vi "4 channel - main interface.vi"() -> ()   [LabVIEW 2023]
uses:
  <vilib>/DAQmx/read.llb/DAQmx Read (Digital 1D Bool 1Chan 1Samp).vi
  <vilib>/DAQmx/create/channels.llb/DAQmx Create Channel (DI-Digital Input).vi
  Shared variables/exp.list.vi
  Shared variables/log.list.vi
  <vilib>/DAQmx/miscellaneous.llb/DAQmx Fill In Error Info.vi
  Shared variables/log.lvlib
panel:
  in  "main interface":T1(tab)
  in  "stop":bool
  in  "Manual control":bool
  in  "Channel":i8=1
  in  "Status":T2(ring)
  out "Current index":i8
  in  "add":bool
  in  "add to exp.list":dbl[](array[numeric])
  in  "Initial index":i8
  out "worker4 times":i8
  out "worker4 entry":i32
  out "worker4 status":dbl(slide) scale=0.0..100.0
  out "worker3 times":i8
  out "worker3 entry":i32
  out "worker3 status":dbl(slide) scale=0.0..100.0
  in  "worker2 on/off":bool
  out "Done":bool
  out "worker2 entry":i32
  out "worker1 entry":i32
  out "worker2 times":i8
  out "worker1 times":i8
  out "worker2 status":dbl(slide) scale=0.0..100.0
  out "worker1 status":dbl(slide) scale=0.0..100.0
  out "wash needle":bool
  out "sensor":bool[](array[boolean])
  in  "worker1 on/off":bool
  in  "worker3 on/off":bool
  in  "worker4 on/off":bool
  out "exp.list":string[][](array[string])
  out "log.list":string[][](array[string])
  # "Designed by @Xian Zheng"
  # "Designed by @Xian Zheng"
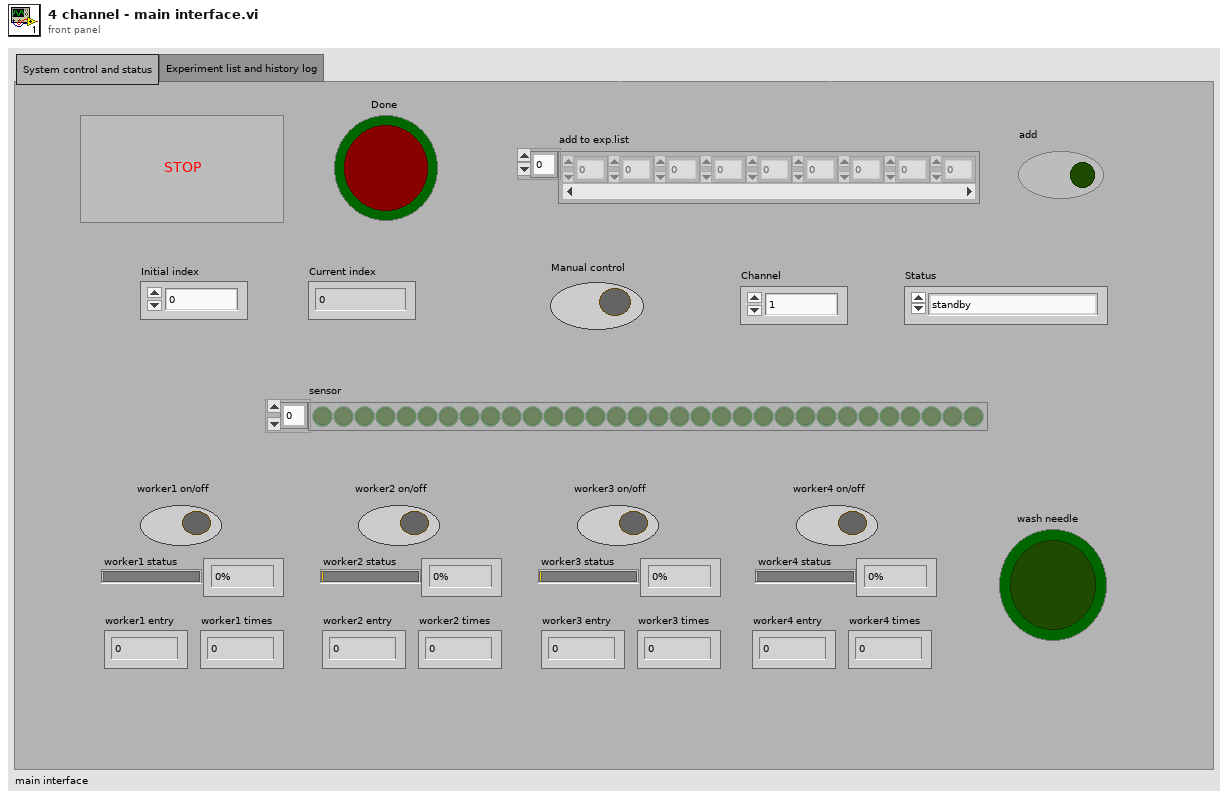
[diagram p1: front panel]
types:
  T1 = enum32{"System control and status", "Experiment list and history log"}
  T2 = enum16{"standby", "prepare droplet", "wash needle", "wash reactor", "wash sample loop", "deliver droplet", "offload product", "oscillate", "transfer product"}
  T3 = enum16{"check", "scan", "index", "read", "add", "write"}
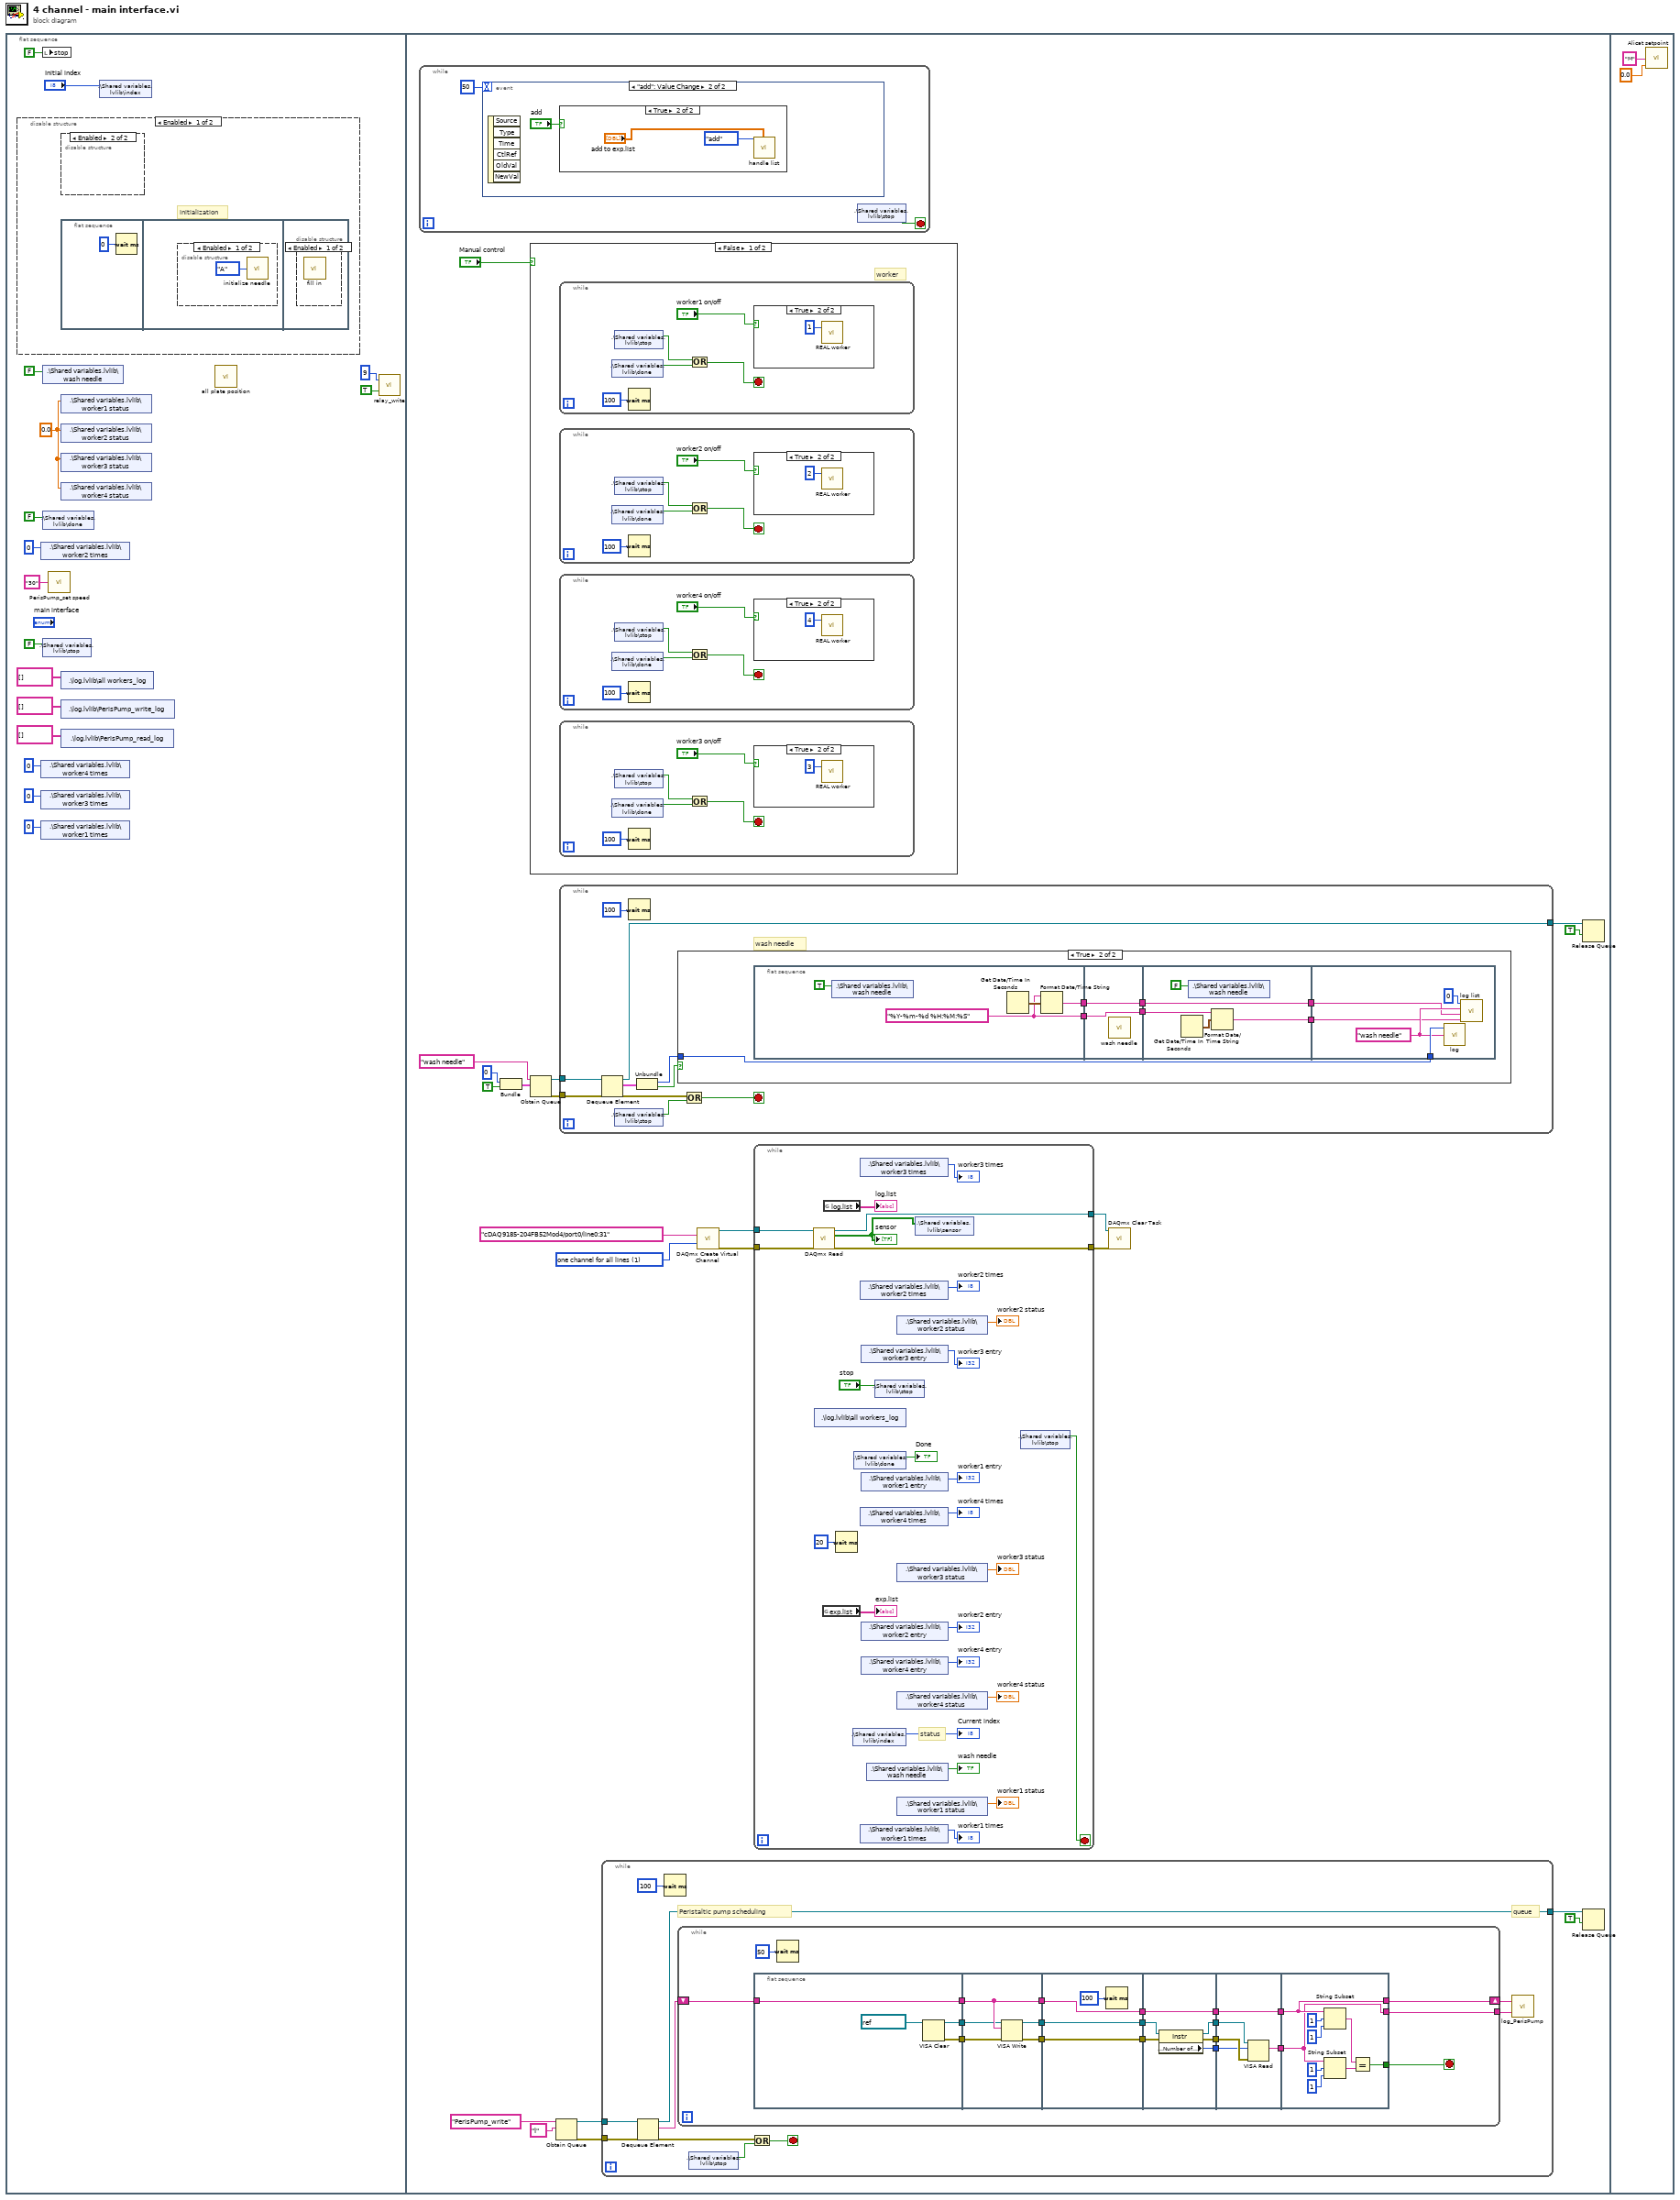
[diagram p0: block diagram]
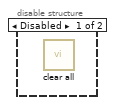
[diagram p2: hidden frame]
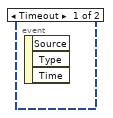
[diagram p6: hidden frame]
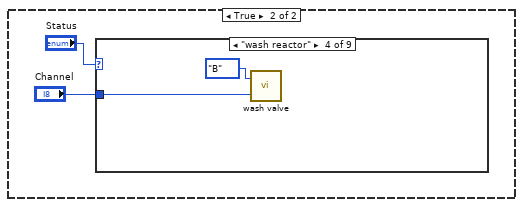
[diagram p13: hidden frame]
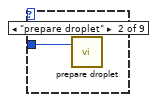
[diagram p15: hidden frame]
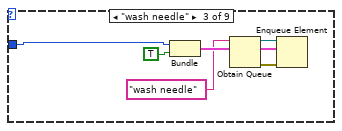
[diagram p16: hidden frame]
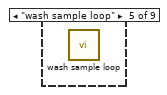
[diagram p17: hidden frame]
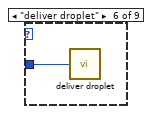
[diagram p18: hidden frame]
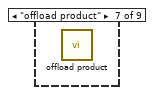
[diagram p19: hidden frame]
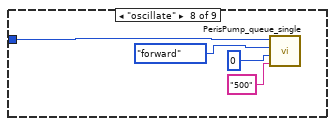
[diagram p20: hidden frame]
diagram:
  n1 = flat-sequence {
    frame #0 {
      w3 = 0.0 ("worker1 status")
      n2 = disable-structure shown="Enabled" {
        frame Enabled {
          # "initialization"
          n3 = disable-structure shown="Enabled" {
            frame Disabled {
              n4 = call "clear all.vi"() -> ()  [unwired: 12 in]
            }
            frame Enabled {
            }
          }
          n5 = flat-sequence {
            frame #0 {
              n6 = Wait (ms)(milliseconds to wait=u32 0) -> ()  [unwired: 1 out]
            }
            frame #1 {
              n7 = disable-structure shown="Enabled" {
                frame Enabled {
                  n8 = call "initialize needle.vi"("Switch to (A/B)"=enum16{"A", "B"}."A") -> ()  [unwired: 1 in]
                }
                frame Disabled {
                }
              }
            }
            frame #2 {
              n9 = disable-structure shown="Enabled" {
                frame Enabled {
                  n10 = call "fill in.vi"() -> ()  [unwired: 12 in]
                }
                frame Disabled {
                }
              }
            }
          }
        }
        frame Disabled {
        }
      }
      n11 = shared-variable ".\\Shared variables.lvlib\\worker2 times"(i8 0 ("worker1 times")) -> ()  [unwired: 1 in, 1 out]
      n12 = shared-variable ".\\Shared variables.lvlib\\worker4 times"(i8 0 ("worker1 times")) -> ()  [unwired: 1 in, 1 out]
      n13 = shared-variable ".\\Shared variables.lvlib\\worker3 times"(i8 0 ("worker1 times")) -> ()  [unwired: 1 in, 1 out]
      n14 = shared-variable ".\\Shared variables.lvlib\\worker1 times"(i8 0 ("worker1 times")) -> ()  [unwired: 1 in, 1 out]
      n15 = local write "stop"(FALSE ("stop")) -> ()
      n16 = shared-variable ".\\Shared variables.lvlib\\wash needle"(FALSE ("wash needle")) -> ()  [unwired: 1 in, 1 out]
      n17 = shared-variable ".\\Shared variables.lvlib\\done"(FALSE ("done")) -> ()  [unwired: 1 in, 1 out]
      n18 = shared-variable ".\\Shared variables.lvlib\\stop"(FALSE ("stop")) -> ()  [unwired: 1 in, 1 out]
      n19 = call "PerisPump_set speed.vi"("Speed (rpm)"="30") -> ()  [unwired: 1 in]
      n20 = shared-variable ".\\Shared variables.lvlib\\worker1 status"(w3) -> ()  [unwired: 1 in, 1 out]
      n21 = shared-variable ".\\Shared variables.lvlib\\worker2 status"(w3) -> ()  [unwired: 1 in, 1 out]
      n22 = shared-variable ".\\Shared variables.lvlib\\worker3 status"(w3) -> ()  [unwired: 1 in, 1 out]
      n23 = shared-variable ".\\Shared variables.lvlib\\worker4 status"(w3) -> ()  [unwired: 1 in, 1 out]
      n24 = shared-variable ".\\log.lvlib\\all workers_log"(string[] [] ("all workers_log")) -> ()  [unwired: 1 in, 1 out]
      n25 = shared-variable ".\\log.lvlib\\PerisPump_write_log"(string[] [] ("PerisPump_write_log")) -> ()  [unwired: 1 in, 1 out]
      n26 = shared-variable ".\\log.lvlib\\PerisPump_read_log"(string[] [] ("PerisPump_write_log")) -> ()  [unwired: 1 in, 1 out]
      n27 = shared-variable ".\\Shared variables.lvlib\\index"("Initial index") -> ()  [unwired: 1 in, 1 out]
      n28 = call "all plate position.vi"() -> ()  [unwired: 3 in, 3 out]
      n29 = call "relay_write.vi"("on/off"=TRUE, "No."=u8 9) -> ()  [unwired: 1 out]
    }
    frame #1 {
      w31 = 1 items=["one channel for each line", "one channel for all lines"] ("line grouping")
      n30 = while {
        stop <- w40 stop-if-true
        n31 = event shown="[1] \"add\": Value Change" {
          selector: _ -> [_ _]
          dyn-events: _ -> [_ _]
          timeout: 50 -> [_ _]
          event Timeout {
            n32 = event-data() -> ()  [unwired: 1 in, 3 out]
          }
          event "add": Value Change {
            n33 = event-data() -> ()  [unwired: 1 in, 6 out]
            n34 = case shown="True" "add" {
              frame False {
              }
              frame True {
                n35 = call "handle list.vi"("operation"=T3."add", "add to list"="add to exp.list") -> ()  [unwired: 14 in, 4 out]
              }
            }
          }
        }
        n36 = shared-variable ".\\Shared variables.lvlib\\stop"() -> (w40:bool)  [unwired: 1 in, 1 out]
      }
      n37 = Bundle(i8 0, TRUE) -> (w21:cluster{i8, bool})  [unwired: 1 in]
      n38 = case shown="False" "Manual control" {
        frame False {
          # "worker"
          n39 = while {
            stop <- w97 stop-if-true
            n40 = shared-variable ".\\Shared variables.lvlib\\done"() -> (w98:bool)  [unwired: 1 in, 1 out]
            n41 = shared-variable ".\\Shared variables.lvlib\\stop"() -> (w99:bool)  [unwired: 1 in, 1 out]
            n42 = Wait (ms)(milliseconds to wait=u32 100) -> ()  [unwired: 1 out]
            n43 = Or(x=w99, y=w98) -> (x .or. y?=w97:bool)
            n44 = case shown="True" "worker1 on/off" {
              frame False {
              }
              frame True {
                n45 = call "REAL worker.vi"("channel"=i8 1) -> ()  [unwired: 2 in, 1 out]
              }
            }
          }
          n46 = while {
            stop <- w92 stop-if-true
            n47 = shared-variable ".\\Shared variables.lvlib\\done"() -> (w94:bool)  [unwired: 1 in, 1 out]
            n48 = shared-variable ".\\Shared variables.lvlib\\stop"() -> (w93:bool)  [unwired: 1 in, 1 out]
            n49 = Wait (ms)(milliseconds to wait=u32 100) -> ()  [unwired: 1 out]
            n50 = Or(x=w93, y=w94) -> (x .or. y?=w92:bool)
            n51 = case shown="True" "worker2 on/off" {
              frame False {
              }
              frame True {
                n52 = call "REAL worker.vi"("channel"=i8 2) -> ()  [unwired: 2 in, 1 out]
              }
            }
          }
          n53 = while {
            stop <- w80 stop-if-true
            n54 = shared-variable ".\\Shared variables.lvlib\\done"() -> (w82:bool)  [unwired: 1 in, 1 out]
            n55 = shared-variable ".\\Shared variables.lvlib\\stop"() -> (w81:bool)  [unwired: 1 in, 1 out]
            n56 = Wait (ms)(milliseconds to wait=u32 100) -> ()  [unwired: 1 out]
            n57 = Or(x=w81, y=w82) -> (x .or. y?=w80:bool)
            n58 = case shown="True" "worker4 on/off" {
              frame False {
              }
              frame True {
                n59 = call "REAL worker.vi"("channel"=i8 4) -> ()  [unwired: 2 in, 1 out]
              }
            }
          }
          n60 = while {
            stop <- w86 stop-if-true
            n61 = shared-variable ".\\Shared variables.lvlib\\done"() -> (w88:bool)  [unwired: 1 in, 1 out]
            n62 = shared-variable ".\\Shared variables.lvlib\\stop"() -> (w87:bool)  [unwired: 1 in, 1 out]
            n63 = Wait (ms)(milliseconds to wait=u32 100) -> ()  [unwired: 1 out]
            n64 = Or(x=w87, y=w88) -> (x .or. y?=w86:bool)
            n65 = case shown="True" "worker3 on/off" {
              frame False {
              }
              frame True {
                n66 = call "REAL worker.vi"("channel"=i8 3) -> ()  [unwired: 2 in, 1 out]
              }
            }
          }
        }
        frame True {
          n67 = case shown="\"wash reactor\"" "Status" {
            tunnel: "Channel" -> [_ w104 w108 w112 _ w113 _ w117 w118]
            frame "standby", Default {
            }
            frame "prepare droplet" {
              n68 = call "prepare droplet.vi"("channel"=w104) -> ()  [unwired: 3 in]
            }
            frame "wash needle" {
              n69 = Bundle("Channel"=w108, TRUE) -> (w106:cluster{"Channel":i8, bool})  [unwired: 1 in]
              n70 = Obtain Queue(name (unnamed)="wash needle", element data type=w106) -> (queue out=w110:refnum<queue>, error out=w109:errorcluster)  [unwired: 3 in, 1 out]
              n71 = Enqueue Element(queue=w110, element=w106, error in (no error)=w109) -> ()  [unwired: 1 in, 3 out]
            }
            frame "wash reactor" {
              n72 = call "wash valve.vi"("channel"=w112, "Switch to position (A/B)"=enum16{"A", "B"}."B") -> ()  [unwired: 1 in]
            }
            frame "wash sample loop" {
              n73 = call "wash sample loop.vi"() -> ()  [unwired: 12 in]
            }
            frame "deliver droplet" {
              n74 = call "deliver droplet.vi"("channel"=w113) -> ()  [unwired: 1 in]
            }
            frame "offload product" {
              n75 = call "offload product.vi"() -> ()  [unwired: 12 in]
            }
            frame "oscillate" {
              n76 = call "PerisPump_queue_single.vi"("Step"="500", "Time/min"=0, "First step"=enum16{"forward", "backward"}."forward", "Address"=w117) -> ()  [unwired: 7 in, 1 out]
            }
            frame "transfer product" {
              n77 = call "transfer product.vi"("channel"=w118) -> ()  [unwired: 1 in]
            }
          }
        }
      }
      n78 = Obtain Queue(name (unnamed)="wash needle", element data type=w21) -> (queue out=w24:refnum<queue>, error out=w25:errorcluster)  [unwired: 3 in, 1 out]
      n79 = Obtain Queue(name (unnamed)="PerisPump_write", element data type="Ì" ("string")) -> (queue out=w37:refnum<queue>, error out=w38:errorcluster)  [unwired: 3 in, 1 out]
      n80 = while {
        tunnel: w25 -> [w53]
        tunnel: w24 -> [w49]
        tunnel: [w45] -> w19
        stop <- w50 stop-if-true
        # "wash needle"
        n81 = Dequeue Element(queue=w49, error in (no error)=w53) -> (queue out=w45:refnum<queue>, element=w48:cluster{i8, bool}, error out=w51:errorcluster)  [unwired: 1 in, 1 out]
        n82 = shared-variable ".\\Shared variables.lvlib\\stop"() -> (w52:bool)  [unwired: 1 in, 1 out]
        n83 = Wait (ms)(milliseconds to wait=u32 100) -> ()  [unwired: 1 out]
        n84 = Unbundle(w48) -> (w46:i8, w47:bool)
        n85 = case shown="True" w47 {
          tunnel: w46 -> [_ w57]
          frame False {
          }
          frame True {
            n86 = flat-sequence {
              tunnel: [w63] -> w60
              tunnel: [w62] -> w59
              tunnel: [w67] -> w56
              tunnel: w60 -> [w67]
              tunnel: [w66] -> w55
              tunnel: w59 -> [w66]
              tunnel: [w71] -> w61
              tunnel: w56 -> [w71]
              tunnel: w55 -> [w69]
              tunnel: [w68] -> w58
              tunnel: w57 -> [w77]
              tunnel: w61 -> [w74]
              tunnel: w58 -> [w73]
              frame #0 {
                w62 = "%Y-%m-%d %H:%M:%S" ("time format string (%c)")
                n87 = shared-variable ".\\Shared variables.lvlib\\wash needle"(TRUE ("wash needle")) -> ()  [unwired: 1 in, 1 out]
                n88 = Get Date/Time In Seconds() -> (seconds since 1Jan1904=w64:timestamp)
                n89 = Format Date/Time String(time format string (%c)=w62, seconds (now)=w64) -> (date/time string=w63:string)  [unwired: 1 in]
              }
              frame #1 {
                n90 = call "wash needle.vi"() -> ()  [unwired: 12 in]
              }
              frame #2 {
                n91 = Get Date/Time In Seconds() -> (seconds since 1Jan1904=w70:timestamp)
                n92 = shared-variable ".\\Shared variables.lvlib\\wash needle"(FALSE ("wash needle")) -> ()  [unwired: 1 in, 1 out]
                n93 = Format Date/Time String(time format string (%c)=w69, seconds (now)=w70) -> (date/time string=w68:string)  [unwired: 1 in]
              }
              frame #3 {
                w75 = "wash needle" ("input string")
                n94 = call "log.vi"("worker"=w77, "input string"=w75) -> ()  [unwired: 6 in, 3 out]
                n95 = call "log list.vi"("end"=w73, "start"=w74, "operaton"=w75, "worker"=i8 0) -> ()  [unwired: 7 in, 1 out]
              }
            }
          }
        }
        n96 = Or(x=w51, y=w52) -> (x .or. y?=w50:bool)
      }
      n97 = while {
        tunnel: w37 -> [w153]
        tunnel: w38 -> [w152]
        tunnel: [w149] -> w39
        stop <- w150 stop-if-true
        # "Peristaltic pump scheduling"
        # "queue"
        n98 = Dequeue Element(queue=w153, error in (no error)=w152) -> (queue out=w149:refnum<queue>, element=w146:string, error out=w148:errorcluster)  [unwired: 1 in, 1 out]
        n99 = Wait (ms)(milliseconds to wait=u32 100) -> ()  [unwired: 1 out]
        n100 = while {
          tunnel: [w166] -> w144
          shift-right: [w167] -> w145
          shift-left: w146 -> [w165]
          stop <- w164 stop-if-true
          n101 = flat-sequence {
            tunnel: w165 -> [w177]
            tunnel: [w177] -> w157
            tunnel: [w175] -> w156
            tunnel: [w174] -> w155
            tunnel: [w180] -> w163
            tunnel: [w182] -> w161
            tunnel: [w181] -> w159
            tunnel: w157 -> [w180]
            tunnel: w156 -> [w179]
            tunnel: w155 -> [w178]
            tunnel: w163 -> [w186]
            tunnel: [w186] -> w162
            tunnel: w161 -> [w185]
            tunnel: [w185] -> w160
            tunnel: w159 -> [w184]
            tunnel: [w184] -> w158
            tunnel: w162 -> [w192]
            tunnel: w160 -> [w191]
            tunnel: [w192] -> w173
            tunnel: [w190] -> w172
            tunnel: [w189] -> w171
            tunnel: w158 -> [w188]
            tunnel: [w187] -> w170
            tunnel: w173 -> [w197]
            tunnel: w172 -> [w195]
            tunnel: w171 -> [w196]
            tunnel: w170 -> [w193]
            tunnel: [w197] -> w169
            tunnel: [w194] -> w168
            tunnel: [w201] -> w166
            tunnel: [w204] -> w167
            tunnel: w169 -> [w204]
            tunnel: w168 -> [w201]
            tunnel: [w198] -> w164
            frame #0 {
              n102 = VISA Clear(VISA resource name=refnum<visa-resource-name> "COM3") -> (VISA resource name out=w175:refnum<visa-resource-name>, error out=w174:errorcluster)  [unwired: 1 in]
            }
            frame #1 {
              n103 = VISA Write(VISA resource name=w179, write buffer=w180, error in (no error)=w178) -> (VISA resource name out=w182:refnum<visa-resource-name>, error out=w181:errorcluster)  [unwired: 1 out]
            }
            frame #2 {
              n104 = Wait (ms)(milliseconds to wait=u32 100) -> ()  [unwired: 1 out]
            }
            frame #3 {
              n105 = property class="Instr"(reference=w191, error in=w188) -> (reference out=w190:refnum<visa-resource-name>, error out=w189:errorcluster, "Serial Settings:Number of Bytes at Serial Port"=w187:u32)
            }
            frame #4 {
              n106 = VISA Read(VISA resource name=w195, byte count=w193, error in (no error)=w196) -> (read buffer=w194:string)  [unwired: 3 out]
            }
            frame #5 {
              n107 = String Subset(string=w204, offset (0)=1, length (rest)=1 ("length (rest)")) -> (substring=w199:string)
              n108 = String Subset(string=w201, offset (0)=1, length (rest)=1 ("length (rest)")) -> (substring=w200:string)
              n109 = Equal?(x=w199, y=w200) -> (x = y?=w198:bool)
            }
          }
          n110 = Wait (ms)(milliseconds to wait=u32 50) -> ()  [unwired: 1 out]
        }
        n111 = shared-variable ".\\Shared variables.lvlib\\stop"() -> (w147:bool)  [unwired: 1 in, 1 out]
        n112 = Or(x=w148, y=w147) -> (x .or. y?=w150:bool)
        n113 = call "log_PerisPump.vi"("read string"=w144, "write string"=w145) -> ()  [unwired: 2 out]
      }
      n114 = call-poly <vilib>:"DAQmx Create Virtual Channel.vi"("lines"=tag "cDAQ9185-204FB52Mod4/port0/line0:31", "line grouping"=w31) -> ("task out"=w30:refnum<k21>, "error out"=w29:errorcluster)  [unwired: 12 in]
      n115 = while {
        tunnel: w30 -> [w139]
        tunnel: w29 -> [w138]
        tunnel: [w136] -> w28
        tunnel: [w135] -> w27
        stop <- w141 stop-if-true
        # "status"
        n116 = call-poly <vilib>:"DAQmx Read.vi"("task/channels in"=w139, "error in"=w138) -> ("task out"=w135:refnum<k21>, "data"=w137:bool[], "error out"=w136:errorcluster)  [unwired: 11 in]
        "sensor" <- w137
        n117 = shared-variable ".\\log.lvlib\\all workers_log"() -> ()  [unwired: 1 in, 2 out]
        n118 = global read "exp.list.vi" "exp.list"() -> (→"exp.list":string[][])
        n119 = global read "log.list.vi" "log.list"() -> (→"log.list":string[][])
        n120 = Wait (ms)(milliseconds to wait=u32 20) -> ()  [unwired: 1 out]
        n121 = shared-variable ".\\Shared variables.lvlib\\index"() -> (→"Current index":i8)  [unwired: 1 in, 1 out]
        n122 = shared-variable ".\\Shared variables.lvlib\\done"() -> (→"Done":bool)  [unwired: 1 in, 1 out]
        n123 = shared-variable ".\\Shared variables.lvlib\\worker3 times"() -> (→"worker3 times":i8)  [unwired: 1 in, 1 out]
        n124 = shared-variable ".\\Shared variables.lvlib\\worker2 times"() -> (→"worker2 times":i8)  [unwired: 1 in, 1 out]
        n125 = shared-variable ".\\Shared variables.lvlib\\worker4 times"() -> (→"worker4 times":i8)  [unwired: 1 in, 1 out]
        n126 = shared-variable ".\\Shared variables.lvlib\\worker1 times"() -> (→"worker1 times":i8)  [unwired: 1 in, 1 out]
        n127 = shared-variable ".\\Shared variables.lvlib\\worker3 entry"() -> (→"worker3 entry":i32)  [unwired: 1 in, 1 out]
        n128 = shared-variable ".\\Shared variables.lvlib\\worker1 entry"() -> (→"worker1 entry":i32)  [unwired: 1 in, 1 out]
        n129 = shared-variable ".\\Shared variables.lvlib\\worker2 entry"() -> (→"worker2 entry":i32)  [unwired: 1 in, 1 out]
        n130 = shared-variable ".\\Shared variables.lvlib\\worker4 entry"() -> (→"worker4 entry":i32)  [unwired: 1 in, 1 out]
        n131 = shared-variable ".\\Shared variables.lvlib\\wash needle"() -> (→"wash needle":bool)  [unwired: 1 in, 1 out]
        n132 = shared-variable ".\\Shared variables.lvlib\\stop"("stop") -> ()  [unwired: 1 in, 1 out]
        n133 = shared-variable ".\\Shared variables.lvlib\\worker2 status"() -> (→"worker2 status":dbl)  [unwired: 1 in, 1 out]
        n134 = shared-variable ".\\Shared variables.lvlib\\worker3 status"() -> (→"worker3 status":dbl)  [unwired: 1 in, 1 out]
        n135 = shared-variable ".\\Shared variables.lvlib\\worker4 status"() -> (→"worker4 status":dbl)  [unwired: 1 in, 1 out]
        n136 = shared-variable ".\\Shared variables.lvlib\\worker1 status"() -> (→"worker1 status":dbl)  [unwired: 1 in, 1 out]
        n137 = shared-variable ".\\Shared variables.lvlib\\sensor"(w137) -> ()  [unwired: 1 in, 1 out]
        n138 = shared-variable ".\\Shared variables.lvlib\\stop"() -> (w141:bool)  [unwired: 1 in, 1 out]
      }
      n139 = call <vilib>:"DAQmx Clear Task.vi"("task in"=w27, "error in"=w28) -> ()  [unwired: 13 in, 1 out]
      n140 = Release Queue(queue=w19, force destroy? (F)=TRUE) -> ()  [unwired: 1 in, 3 out]
      n141 = Release Queue(queue=w39, force destroy? (F)=TRUE) -> ()  [unwired: 1 in, 3 out]
    }
    frame #2 {
      n142 = call "Alicat setpoint.vi"("Setpoint"=0.0, "Unit ID"="M") -> ()  [unwired: 3 in]
    }
  }
